vi "Entry.vi"(8 "error in (no error)":errorcluster, 11 "New State":refnum<class "Completed Command.lvclass">) -> (0 "error out":errorcluster, 3 "State out":refnum<class "Completed Command.lvclass">)   [LabVIEW 2013, in "Command Actor.lvlib" / "Completed Command.lvclass"]
doc: "This is an abstract method. Override this method to define the behavior when you enter the state."
uses:
  Completed Command.lvclass
  <vilib>/ActorFramework/Actor/Actor.lvclass/Actor.ctl
  Command States.lvclass
  <vilib>/ActorFramework/Message Enqueuer/Message Enqueuer.lvclass/Message Enqueuer.ctl
  <vilib>/ActorFramework/Message Enqueuer/Enqueue.vi
  <vilib>/ActorFramework/Message Priority Queue/Priority Enqueue.vi
  Command Actor Messages/Completed Msg/Completed Msg.lvclass
  <vilib>/ActorFramework/Actor/Actor.lvclass
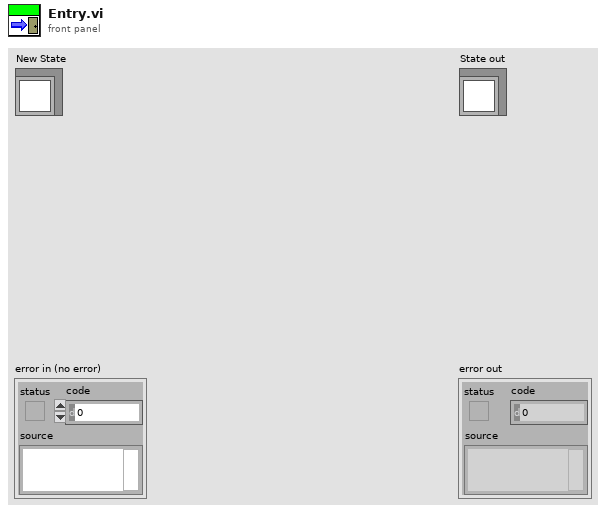
[diagram p1: front panel]
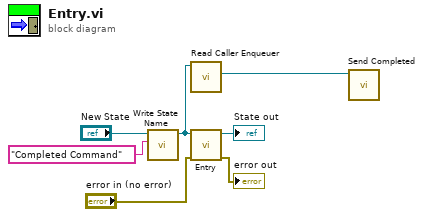
[diagram p0: block diagram]
diagram:
  n1 = call-dynamic "Write State Name.vi"("State Name"="Completed Command", "Command States in"="New State") -> ("Command States out"=w2:refnum<class "Completed Command.lvclass">)  [unwired: 8 in, 1 out]
  n2 = call <vilib>:"Read Caller Enqueuer.vi"("Actor"=w2) -> ("Caller Enqueuer"=w1:refnum<class "Message Enqueuer.lvclass">)  [unwired: 10 in]
  n3 = call-parent "Entry.vi"("error in (no error)"="error in (no error)", "New State"=w2) -> ("error out"=→"error out":errorcluster, "State out"=→"State out":refnum<class "Completed Command.lvclass">)  [unwired: 8 in]
  n4 = call "Send Completed.vi"("Message Enqueuer"=w1) -> ()  [unwired: 9 in, 2 out]
